vi "2015_HashSupport.vi"(8 "error in (no error)":errorcluster) -> (0 "error out":errorcluster)   [LabVIEW 2013]
uses:
  source/Cron.Jenkins/Cron.Jenkins.lvclass/Cron.Jenkins.ctl
  source/Cron.Jenkins/Write Job Name.vi
  <vilib>/addons/_JKI Toolkits/Caraya/classes/Assert/Assert True.vi
  source/Cron/Create Cron Job.vi
  source/Cron/Compute Next Cron.vi
  source/Cron.Jenkins/Cron.Jenkins.lvclass
  <vilib>/addons/_JKI Toolkits/Caraya/classes/Test/Test.lvclass
  <vilib>/addons/_JKI Toolkits/Caraya/classes/Assert/Assert.lvclass
  source/openCron.lvlib
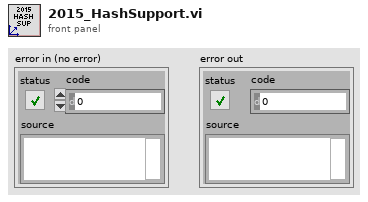
[diagram p1: front panel]
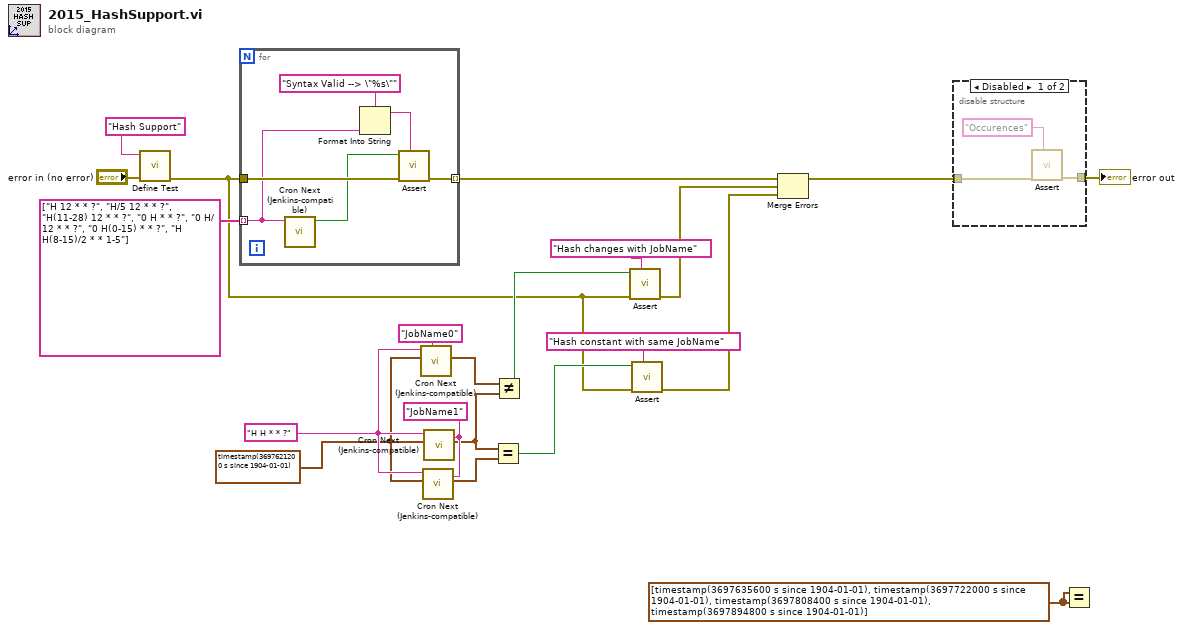
[diagram p0: block diagram]
diagram:
  w11 = "JobName1" ("Expression")
  w9 = "H H * * ?" ("Expression")
  w18 = timestamp[] [timestamp(3697635600 s since 1904-01-01), timestamp(3697722000 s since 1904-01-01), timestamp(3697808400 s since 1904-01-01), timestamp(3697894800 s since 1904-01-01)]
  w8 = timestamp(3697621200 s since 1904-01-01) ("y")
  n1 = call <vilib>:"Define Test.vi"("error in (no error)"="error in (no error)", "Label (VI Title)"="Hash Support") -> ("error out"=w1:errorcluster)  [unwired: 9 in]
  n2 = for {
    tunnel: w1 -> [w27]
    tunnel: [w26] -> w17 mode=indexing
    tunnel: string[] ["H 12 * * ?", "H/5 12 * * ?", "H(11-28) 12 * * ?", "0 H * * ?", "0 H/12 * * ?", "0 H(0-15) * * ?", "H H(8-15)/2 * * 1-5"] -> [w22] mode=indexing
    n3 = call "Cron Next (Jenkins-compatible).vi"("Cron Expression"=w22) -> ("syntax valid?"=w25:bool)  [unwired: 8 in, 2 out]
    n4 = Format Into String(format string="Syntax Valid --> \"%s\"" ("Label (VI Title)"), w22) -> (resulting string=w23:string)  [unwired: 2 in, 1 out]
    n5 = call-poly <vilib>:"Assert.vi"("Label"=w23, "error in (no error)"=w27, "True?"=w25) -> ("error out"=w26:errorcluster)  [unwired: 8 in]
  }
  n6 = call "Cron Next (Jenkins-compatible).vi"("Job Name"="JobName0" ("Expression"), "Reference timestamp (Now)"=w8, "Cron Expression"=w9) -> ("Next Occurence"=w7:timestamp)  [unwired: 6 in, 2 out]
  n7 = call "Cron Next (Jenkins-compatible).vi"("Job Name"=w11, "Reference timestamp (Now)"=w8, "Cron Expression"=w9) -> ("Next Occurence"=w4:timestamp)  [unwired: 6 in, 2 out]
  n8 = call "Cron Next (Jenkins-compatible).vi"("Job Name"=w11, "Reference timestamp (Now)"=w8, "Cron Expression"=w9) -> ("Next Occurence"=w3:timestamp)  [unwired: 6 in, 2 out]
  n9 = Equal?(x=w3, y=w4) -> (x = y?=w2:bool)
  n10 = Not Equal?(x=w7, y=w3) -> (x != y?=w13:bool)
  n11 = call-poly <vilib>:"Assert.vi"("Label"="Hash changes with JobName" ("Label (VI Title)"), "error in (no error)"=w1, "True?"=w13) -> ("error out"=w14:errorcluster)  [unwired: 8 in]
  n12 = call-poly <vilib>:"Assert.vi"("Label"="Hash constant with same JobName" ("Label (VI Title)"), "error in (no error)"=w1, "True?"=w2) -> ("error out"=w5:errorcluster)  [unwired: 8 in]
  n13 = Merge Errors(w17, w14, w5) -> (w16:errorcluster)
  n14 = disable-structure "Diagram Disable Structure" shown="Disabled" {
    disable-tunnel: [w30 w31] -> w21
    disable-tunnel: w16 -> [w28 w31]
    frame Disabled {
      n15 = call-poly <vilib>:"Assert.vi"("Label"="Occurences" ("Label (VI Title)"), "error in (no error)"=w28) -> ("error out"=w30:errorcluster)  [unwired: 9 in]
    }
    frame Enabled {
    }
  }
  "error out" <- w21
  n16 = Equal?(x=w18, y=w18) -> ()  [unwired: 1 out]
